vi "VideoCapture_Probe.vi"(11 "OpenLvVision_OpenCv.lvlib:VideoCapture":refnum<class "VideoCapture.lvclass">) -> (2 "Value String":string, 3 "Pause VI":bool)   [LabVIEW 2020, in "OpenLvVision_OpenCv.lvlib" / "VideoCapture.lvclass"]
uses:
  VideoCapture.lvclass
  C:/Users/lukas/Downloads/OpenLvVision_OpenCv/SourceCode/LabView/OpenLvVision_OpenCv/_LvHelpers/EdvrObject/EdvrObject.lvclass
  _LvHelpers/EdvrObject/EdvrObject.lvclass/EdvrObject.ctl
  _LvHelpers/EdvrObject/EdvrObject.lvclass
panel:
  out "BackendName":string
  out "Open":bool
  out "Reference":u64 format="%.0x"
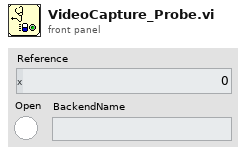
[diagram p1: front panel]
types:
  T1 = typedef "OpenLvVision_OpenCv.lvlib/EdvrObject.lvclass/Edvr.ctl" = refnum<data-value>
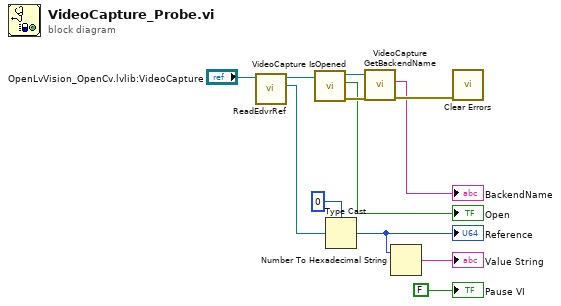
[diagram p0: block diagram]
diagram:
  n1 = call "ReadEdvrRef.vi"("EdvrObject in"="OpenLvVision_OpenCv.lvlib:VideoCapture") -> ("Edvr"=w8:T1, "EdvrObject out"=w7:refnum<class "VideoCapture.lvclass">)  [unwired: 8 in, 1 out]
  n2 = call "VideoCapture IsOpened.vi"("VideoCapture in"=w7) -> ("error out"=w5:errorcluster, "Open"=→"Open":bool, "VideoCapture out"=w6:refnum<class "VideoCapture.lvclass">)  [unwired: 8 in]
  n3 = Type Cast(type=u64 0, x=w8) -> (*(type *) &x=w10:u64)
  "Reference" <- w10
  n4 = call "VideoCapture GetBackendName.vi"("error in (no error)"=w5, "VideoCapture in"=w6) -> ("error out"=w4:errorcluster, "BackendName"=→"BackendName":string)  [unwired: 7 in, 1 out]
  n5 = Number To Hexadecimal String(2:w10) -> (0:→"Value String":string)  [unwired: 1 in]
  n6 = call <vilib>:"Clear Errors.vi"("error in (no error)"=w4) -> ()  [unwired: 5 in, 2 out]
  "Pause VI" <- FALSE
